vi "house_debugOnly.vi"() -> ()   [LabVIEW 2014]
panel:
  out "error out":errorcluster
  out "?":bool
  out "?":bool
  out "?":bool
  out "?":bool
  out "?":bool
  out "?":bool
  out "?":bool
  out "?":bool
  out "?":bool
  out "?":bool
  out "8 wire data":u8
  in  "DAC  1 [V]":dbl min=-5.0 max=5.0
  in  "VISA resource name":refnum<visa-resource-name>
  out "Device ID":string
  in  "Stop Button":bool
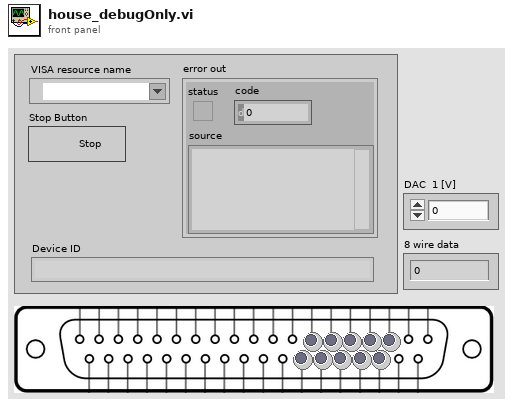
[diagram p1: front panel]
types:
  T1 = cluster{"P1_0":bool, "P1_1":bool, "P1_2":bool, "P1_3":bool, "P1_4":bool, "P1_5":bool, "P1_6":bool, "P1_7":bool, "NC":bool}
  T2 = cluster{"P0_0":bool, "P1_1":bool, "P0_2":bool, "P0_3":bool, "P0_4":bool, "P0_5":bool, "P0_6":bool, "P0_7":bool, "NC":bool}
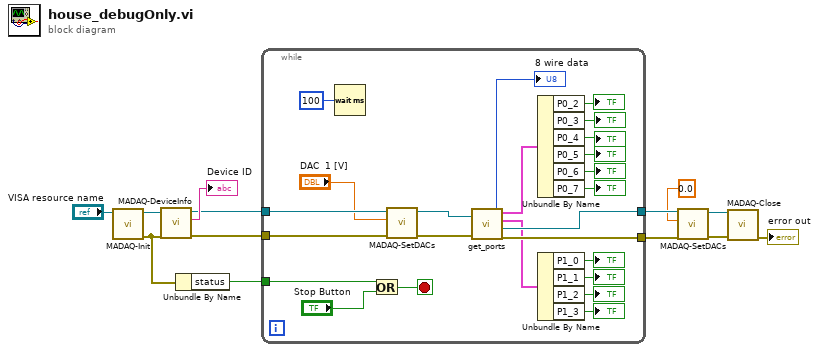
[diagram p0: block diagram]
diagram:
  n1 = call "MADAQ-Init.vi"("VISA resource name"="VISA resource name") -> ("error out"=w3:errorcluster, "VISA resource name out"=w12:refnum<visa-resource-name>)  [unwired: 5 in]
  n2 = call "MADAQ-DeviceInfo.vi"("error in (no error)"=w3, "VISA resource name"=w12) -> ("error out"=w11:errorcluster, "Device ID"=→"Device ID":string, "VISA resource name out"=w9:refnum<visa-resource-name>)  [unwired: 3 in]
  n3 = Unbundle By Name(w3) -> ("status"=w2:bool)
  n4 = while {
    tunnel: w11 -> [w36]
    tunnel: w9 -> [w35]
    tunnel: [w28] -> w7
    tunnel: [w32] -> w8
    tunnel: w2 -> [w30]
    stop <- w31 stop-if-true
    n5 = Wait (ms)(milliseconds to wait=u32 100) -> ()  [unwired: 1 out]
    n6 = Or(x=w30, y="Stop Button") -> (x .or. y?=w31:bool)
    n7 = call "MADAQ-SetDACs.vi"("error in (no error)"=w36, "DAC  1 [V]"="DAC  1 [V]", "VISA resource name"=w35) -> ("error out"=w33:errorcluster, "VISA resource name out"=w34:refnum<visa-resource-name>)  [unwired: 3 in]
    n8 = call "get_ports.vi"("error in (no error)"=w33, "VISA Refnum in"=w34) -> ("error out"=w32:errorcluster, "VISA Refnum out"=w28:refnum<visa-resource-name>, "P1"=w25:T1, "P0"=w20:T2, "data"=→"8 wire data":u8)
    n9 = Unbundle By Name(w20) -> ("P0_2"=→"?":bool, "P0_3"=→"?":bool, "P0_4"=→"?":bool, "P0_5"=→"?":bool, "P0_6"=→"?":bool, "P0_7"=→"?":bool)
    n10 = Unbundle By Name(w25) -> ("P1_0"=→"?":bool, "P1_1"=→"?":bool, "P1_2"=→"?":bool, "P1_3"=→"?":bool)
  }
  n11 = call "MADAQ-SetDACs.vi"("error in (no error)"=w8, "DAC  1 [V]"=0.0, "VISA resource name"=w7) -> ("error out"=w5:errorcluster, "VISA resource name out"=w6:refnum<visa-resource-name>)  [unwired: 3 in]
  n12 = call "MADAQ-Close.vi"("error in (no error)"=w5, "VISA resource name"=w6) -> ("error out"=→"error out":errorcluster)  [unwired: 4 in, 1 out]
